vi "Realsense Cam Connect.vi"(8 "error in (no error)":errorcluster, 11 "Realsense Cam In":refnum<class "Realsense Cam.lvclass">) -> (0 "error out":errorcluster, 1 "init error":string="No Error\rNo Error\rNo Error\rNo Error\rNo Error\rNo Error\rNo Error\rNo Error\rNo Error\rNo Error\rNo Error", 2 "Found?":bool, 3 "Realsense Cam Out":refnum<class "Realsense Cam.lvclass">)   [LabVIEW 2018, in "Realsense Cam.lvclass"]
uses:
  Realsense Cam.lvclass
  Realsense Cam.lvclass/Realsense Cam.ctl
  realsense_wrapper_api/libRealSense3.lvlib
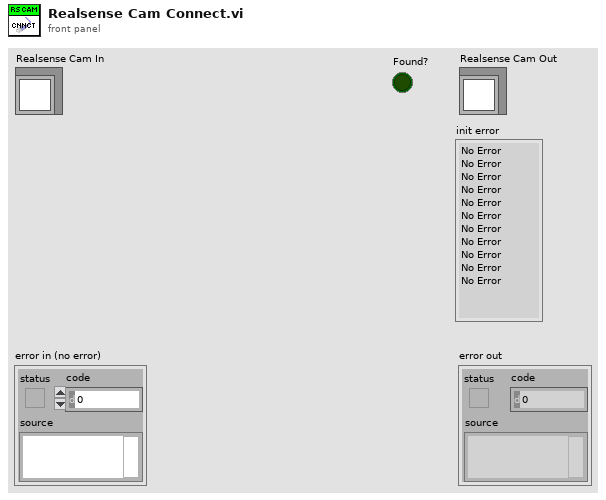
[diagram p1: front panel]
types:
  T1 = cluster{"Depth?":bool, "Left IR?":bool, "Right IR?":bool, "Color?":bool, "RGB Ext.?":bool, "Left IR Unrectified?":bool, "Right IR Unrectified?":bool}
  T2 = cluster{"camera name":string, "camera S/N":string, "F/W":string, "Sensor name":string, "api_version":i32, "rscontext":u64, "device_list":u64, "device count":i32, "Dev out":u64, "sensor_list":u64, "sensor count":i32, "Sensor out":u64}
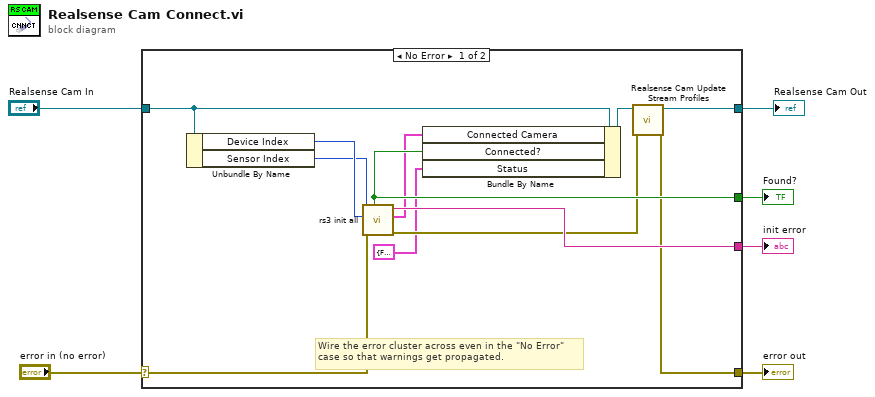
[diagram p0: block diagram]
diagram:
  n1 = case shown="No Error" "error in (no error)" {
    selector: "error in (no error)" -> [w16 w20]
    tunnel: [w9 w20] -> w5
    tunnel: [w8 w19] -> w1
    tunnel: "Realsense Cam In" -> [w14 w19]
    tunnel: [w15 _] -> w4
    tunnel: [w13 _] -> w3
    frame No Error {
      # "Wire the error cluster across even in the \"No Error\"\ncase so that warnings get propagated."
      n2 = Unbundle By Name(w14) -> ("Device Index"=w18:i32, "Sensor Index"=w17:i32)
      n3 = call "rs3 init all.vi"("error in"=w16, "Select Device"=w18, "Select Sensor"=w17) -> ("error out"=w10:errorcluster, "init results"=w12:T2, "init error"=w15:string, "Found RealSense"=w13:bool)  [unwired: 2 in, 3 out]
      n4 = Bundle By Name(cluster=w14, "Connected Camera"=w12, "Connected?"=w13, "Status"=T1 {"Depth?"=FALSE, "Left IR?"=FALSE, "Right IR?"=FALSE, "Color?"=FALSE, "RGB Ext.?"=FALSE, "Left IR Unrectified?"=FALSE, "Right IR Unrectified?"=FALSE} ("Stream Data.Current.Status")) -> (w11:refnum<class "Realsense Cam.lvclass">)
      n5 = call "Realsense Cam Update Stream Profiles.vi"("error in (no error)"=w10, "Realsense Cam in"=w11) -> ("error out"=w9:errorcluster, "Realsense Cam out"=w8:refnum<class "Realsense Cam.lvclass">)  [unwired: 8 in]
    }
    frame Error {
    }
  }
  "error out" <- w5
  "Found?" <- w3
  "init error" <- w4
  "Realsense Cam Out" <- w1
